vi "探头清洗间隔.vi"(7 "校准参数":u16(ring) caption="校准参数：" items=["pH", "DO", "浊度", "电导率", "叶绿素a", "藻密度", "ORP", "DO2"], 8 "error in (no error)":errorcluster caption="错误输入（无错误）", 11 "清扫间隔":u16) -> (0 "error out":errorcluster caption="错误输出")   [LabVIEW 2022 SP3, in "斯坦道多参数.lvlib"]
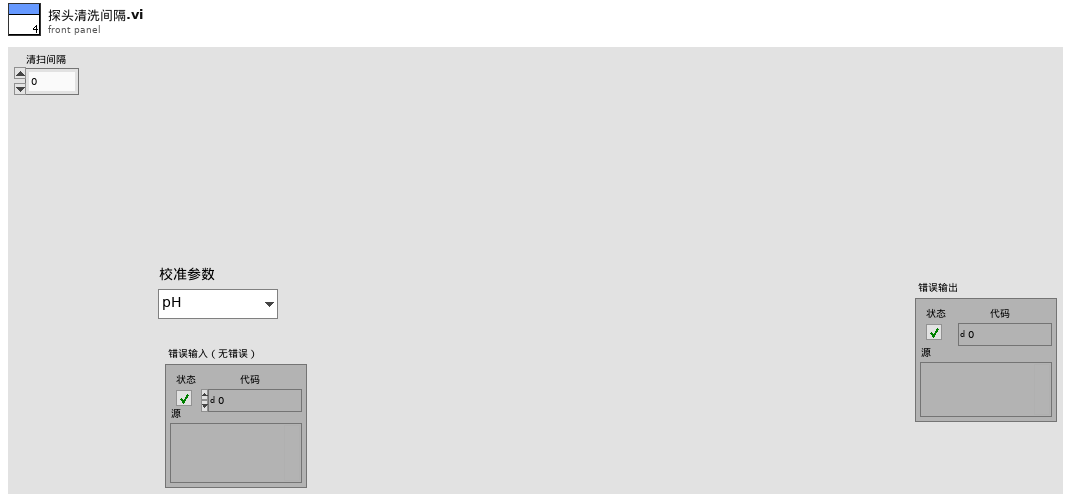
[diagram p1: front panel]
types:
  T1 = typedef "斯坦道多参数.lvlib/探头类型.ctl" = enum16{"禹山", "国弘", "纳清", "STD"}
  T2 = enum16{"NULL", "pH", "Cond", "DO", "Turb", "ORP"}
  T3 = enum16{"null", "pH", "DO", "浊度", "电导率", "叶绿素a", "藻密度"}
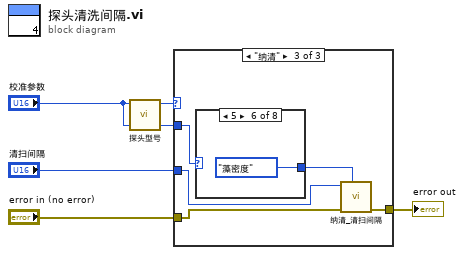
[diagram p0: block diagram]
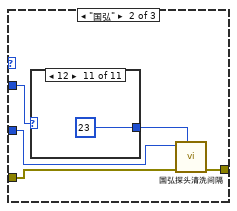
[diagram p3: hidden frame]
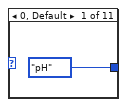
[diagram p4: hidden frame]
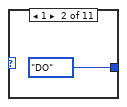
[diagram p5: hidden frame]
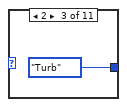
[diagram p6: hidden frame]
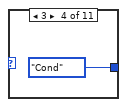
[diagram p7: hidden frame]
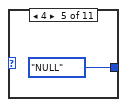
[diagram p8: hidden frame]
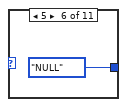
[diagram p9: hidden frame]
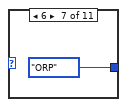
[diagram p10: hidden frame]
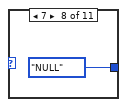
[diagram p11: hidden frame]
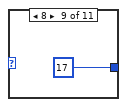
[diagram p12: hidden frame]
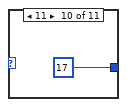
[diagram p13: hidden frame]
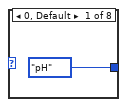
[diagram p14: hidden frame]
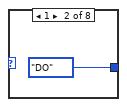
[diagram p15: hidden frame]
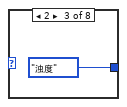
[diagram p16: hidden frame]
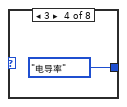
[diagram p17: hidden frame]
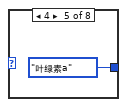
[diagram p18: hidden frame]
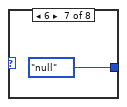
[diagram p19: hidden frame]
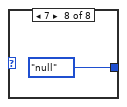
[diagram p20: hidden frame]
diagram:
  n1 = call "探头型号.vi"("校准参数"="校准参数") -> ("探头型号"=w5:T1)  [unwired: 8 in, 2 out]
  n2 = case shown="\"纳清\"" w5 {
    tunnel: "校准参数" -> [_ w11 w27]
    tunnel: "error in (no error)" -> [w6 w10 w25]
    tunnel: [w6 w8 w24] -> w2
    tunnel: "清扫间隔" -> [_ w7 w23]
    frame "禹山", Default {
    }
    frame "国弘" {
      n3 = case shown="12" w11 {
        tunnel: [T2."pH" ("探头") T2."DO" ("探头") T2."Turb" ("探头") T2."Cond" ("探头") T2."NULL" ("探头") T2."NULL" ("探头") T2."ORP" ("探头") T2."NULL" ("探头") 17 ("探头") 17 ("探头") 23 ("探头")] -> w9
        frame 0, Default {
        }
        frame 1 {
        }
        frame 2 {
        }
        frame 3 {
        }
        frame 4 {
        }
        frame 5 {
        }
        frame 6 {
        }
        frame 7 {
        }
        frame 8 {
        }
        frame 11 {
        }
        frame 12 {
        }
      }
      n4 = call "国弘探头清洗间隔.vi"("探头"=w9, "error in (no error)"=w10, "清洗间隔"=w7) -> ("error out"=w8:errorcluster)  [unwired: 7 in, 1 out]
    }
    frame "纳清" {
      n5 = case shown="5" w27 {
        tunnel: [T3."pH" ("探头") T3."DO" ("探头") T3."浊度" ("探头") T3."电导率" ("探头") T3."叶绿素a" ("探头") T3."藻密度" ("探头") T3."null" ("探头") T3."null" ("探头")] -> w26
        frame 0, Default {
        }
        frame 1 {
        }
        frame 2 {
        }
        frame 3 {
        }
        frame 4 {
        }
        frame 5 {
        }
        frame 6 {
        }
        frame 7 {
        }
      }
      n6 = call "纳清_清扫间隔.vi"("探头"=w26, "error in (no error)"=w25, "清扫间隔"=w23) -> ("error out"=w24:errorcluster)  [unwired: 8 in]
    }
  }
  "error out" <- w2
